vi "替换询问.vi"(11 "TDMS/TDM File":path) -> (3 "替换":bool)   [LabVIEW 2018]
uses:
  <vilib>/regexp/Match Regular Expression.xnode
panel:
  out "String":string
  in  "单选":bool
  in  "否":bool
  in  "是":bool
  # "文件已存在，是否替换？"
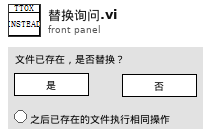
[diagram p1: front panel]
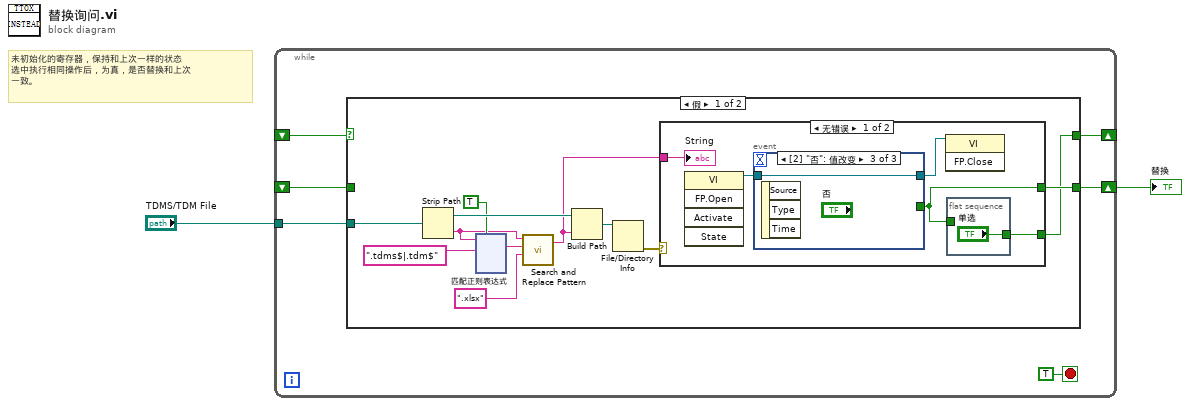
[diagram p0: block diagram]
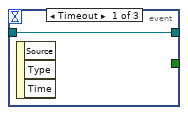
[diagram p2: hidden frame]
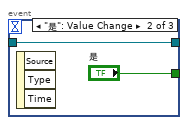
[diagram p3: hidden frame]
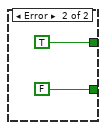
[diagram p4: hidden frame]
diagram:
  # "未初始化的寄存器，保持和上次一样的状态\n选中执行相同操作后，为真，是否替换和上次\n一致。"
  n1 = while {
    tunnel: "TDMS/TDM File" -> [w8]
    shift-right: [w7] -> w1
    shift-left: _ -> [w4]
    shift-right: [w5] -> _
    shift-left: _ -> [w3]
    stop <- TRUE stop-if-true
    n2 = case shown="假" w3 {
      selector: w3 -> [_ w147]
      tunnel: w8 -> [w19 _]
      tunnel: [w15 w148] -> w7
      tunnel: [w10 w147] -> w5
      tunnel: w4 -> [_ w148]
      frame False {
        n3 = Strip Path(path=w19) -> (stripped path=w18:path, name=w11:string)
        n4 = xnode "匹配正则表达式"("输入字符串"=w11, "正则表达式"=".tdms$|.tdm$" ("regular expression (\"\")"), "忽略大小写？(F)"=TRUE) -> ("所有匹配"=w13:string)  [unwired: 3 in, 4 out]
        n5 = call <vilib>:"Search and Replace Pattern.vi"("string"=w11, "regular expression (\"\")"=w13, "replace string (\"\")"=".xlsx" ("replace string (\"\")")) -> ("result string"=w9:string)  [unwired: 2 in, 1 out]
        n6 = Build Path(base path=w18, name or relative path=w9) -> (appended path=w17:path)
        n7 = File/Directory Info(path=w17) -> (error out=w16:errorcluster)  [unwired: 1 in, 6 out]
        n8 = case shown="无错误" w16 {
          tunnel: [w135 TRUE] -> w15
          tunnel: [w137 FALSE ("单选")] -> w10
          tunnel: w9 -> [w136 _]
          frame No Error {
            n9 = invoke class="VI" method="FP.Open"() -> (reference out=w139:refnum<vi>)  [unwired: 5 in, 4 out]
            n10 = event shown="[2] \"否\": 值改变" {
              selector: _ -> [_ _ _]
              dyn-events: _ -> [_ _ _]
              timeout: _ -> [_ _ _]
              tunnel: w139 -> [w141 w143 w144]
              tunnel: [w141 w143 w144] -> w138
              tunnel: [_ "是" _] -> w135
              event Timeout {
                n11 = event-data() -> ()  [unwired: 1 in, 3 out]
              }
              event "是": Value Change {
                n12 = event-data() -> ()  [unwired: 1 in, 3 out]
              }
              event "否": Value Change {
                n13 = event-data() -> ()  [unwired: 1 in, 3 out]
              }
            }
            n14 = invoke class="VI" method="FP.Close"(reference=w138) -> ()  [unwired: 2 in, 3 out]
            n15 = flat-sequence {
              tunnel: ["单选"] -> w137
              tunnel: w135 -> [_]
              frame #0 {
              }
            }
            "String" <- w136
          }
          frame Error {
          }
        }
      }
      frame True {
        # "之后的和上次一样"
      }
    }
  }
  "替换" <- w1
